vi "Robust Update.vi"(5 "condition":string, 7 "data":variant, 8 "error in (no error)":errorcluster, 9 "columns":string[](array[string])=["beh_stop_time"], 10 "table":string="behavior_traces ", 11 "AcquistionObject.lvclass":refnum<class "AcquistionObject.lvclass">) -> (0 "error out":errorcluster, 3 "AcquistionObject out":refnum<class "AcquistionObject.lvclass">)   [LabVIEW 2011, in "AcquistionObject.lvclass"]
uses:
  AcquistionObject.lvclass
  <vilib>/addons/database/NI_Database_API.lvlib
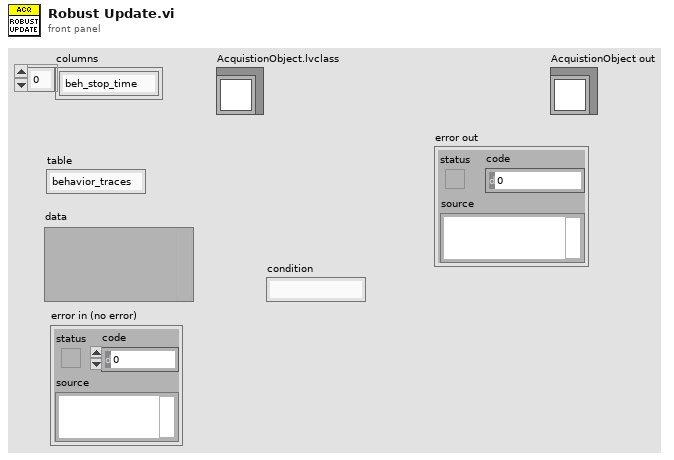
[diagram p1: front panel]
types:
  T1 = typedef "NI_Database_API.lvlib/Conn ObjectReference.ctl" = refnum<k1>
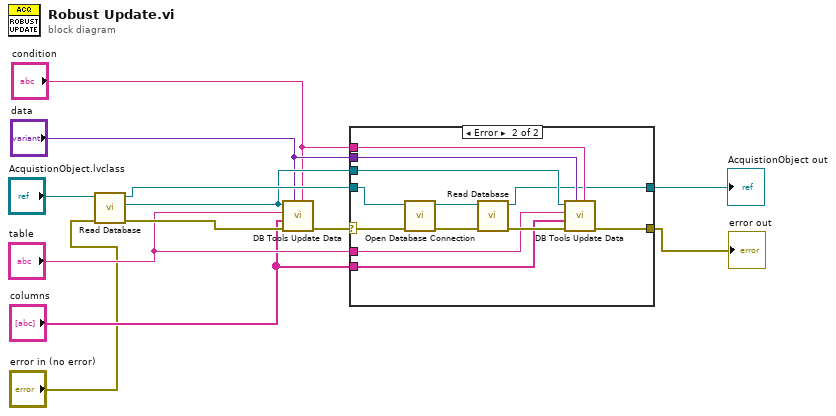
[diagram p0: block diagram]
diagram:
  n1 = call-dynamic "Read Database.vi"("error in (no error)"="error in (no error)", "AcquistionObject in"="AcquistionObject.lvclass") -> ("error out"=w11:errorcluster, "reference"=w6:T1, "AcquistionObject out"=w9:refnum<class "AcquistionObject.lvclass">)  [unwired: 7 in]
  n2 = call <vilib>:"DB Tools Update Data.vi"("condition"="condition", "data"="data", "error in (no error)"=w11, "columns"="columns", "table"="table", "connection reference"=w6) -> ("error out"=w10:errorcluster)  [unwired: 4 in, 1 out]
  n3 = case shown="Error" w10 {
    selector: w10 -> [w13 w26]
    tunnel: w9 -> [w14 w25]
    tunnel: "table" -> [_ w21]
    tunnel: "columns" -> [_ w20]
    tunnel: w6 -> [_ w19]
    tunnel: "data" -> [_ w18]
    tunnel: "condition" -> [_ w17]
    tunnel: [w13 w16] -> w2
    tunnel: [w14 w15] -> w3
    frame No Error {
    }
    frame Error {
      n4 = call-dynamic "Open Database Connection.vi"("error in (no error)"=w26, "AcquistionObject in"=w25) -> ("error out"=w23:errorcluster, "AcquistionObject out"=w24:refnum<class "AcquistionObject.lvclass">)  [unwired: 8 in]
      n5 = call-dynamic "Read Database.vi"("error in (no error)"=w23, "AcquistionObject in"=w24) -> ("error out"=w22:errorcluster, "AcquistionObject out"=w15:refnum<class "AcquistionObject.lvclass">)  [unwired: 7 in, 1 out]
      n6 = call <vilib>:"DB Tools Update Data.vi"("condition"=w17, "data"=w18, "error in (no error)"=w22, "columns"=w20, "table"=w21, "connection reference"=w19) -> ("error out"=w16:errorcluster)  [unwired: 4 in, 1 out]
    }
  }
  "AcquistionObject out" <- w3
  "error out" <- w2
